vi "Error 5002 - Invalid Digital IO Channel Number.vi"() -> (0 "error out":errorcluster)   [LabVIEW 2021]
doc: "Error, channel number is invalid."
uses:
  <vilib>/Utility/error.llb/Error Cluster From Error Code.vi
  <vilib>/ErrorRing/Error Ring.xnode
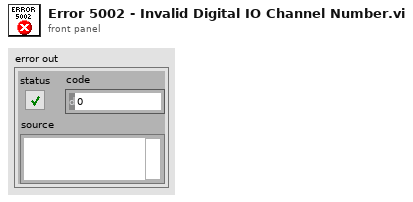
[diagram p1: front panel]
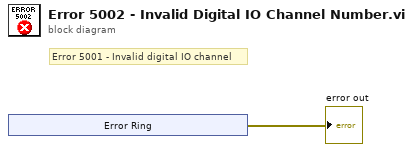
[diagram p0: block diagram]
diagram:
  # "Error 5001 - Invalid digital IO channel"
  n1 = xnode "Error Ring"() -> ("error out"=→"error out":errorcluster)
